vi "ReadSpetroFile.vi"(1 "本次文件名":string) -> ()   [LabVIEW 2018]
uses:
  Init/AllPath.vi
  <vilib>/Utility/file.llb/Read Delimited Spreadsheet (string).vi
  HistoryFile.vi
panel:
  out "波形":cluster{"数组":dbl[], "数组":dbl[]}
  out "脉宽":string
  out "中心波长":string
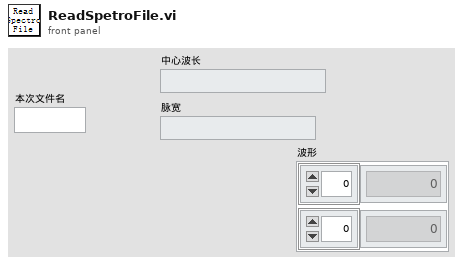
[diagram p1: front panel]
types:
  T1 = cluster{"能量/功率":path, " 示波器":path, " 光谱仪":path, "偏振":path, "近远场":cluster{" 近场图片":path, " 远场图片":path, "发散角数据":path}, "参数":path, " 基路径":path, "文件名信息":path, "输出模板路径":path, "输出报告路径":path, "位置信息路径":path}
  T2 = cluster{"中心波长":string, " 谱宽":string, " 中心波长Uint":string, " 谱宽 Uint":string, "波形":cluster{"数组":dbl[], "数组":dbl[]}}
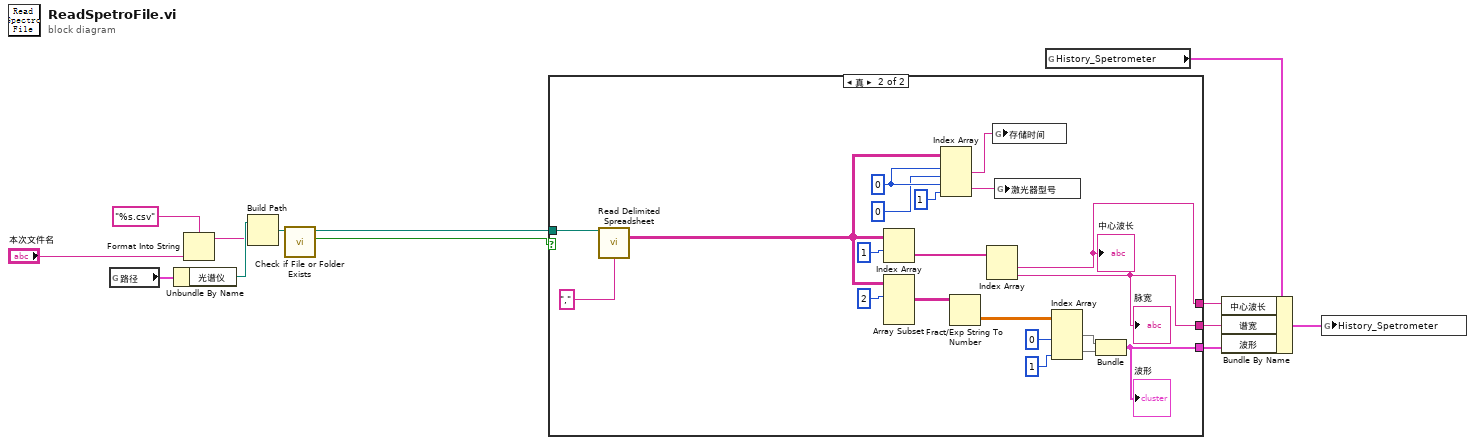
[diagram p0: block diagram]
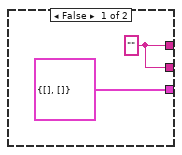
[diagram p2: hidden frame]
diagram:
  n1 = global read "AllPath.vi" "路径"() -> (w13:T1)
  n2 = Unbundle By Name(w13) -> ("光谱仪"=w12:path)
  n3 = Format Into String(format string="%s.csv" ("格式字符串"), "本次文件名") -> (resulting string=w9:string)  [unwired: 2 in, 1 out]
  n4 = Build Path(base path=w12, name or relative path=w9) -> (appended path=w3:path)
  n5 = call <vilib>:"Check if File or Folder Exists.vi"("path"=w3) -> ("file or folder exists?"=w1:bool, "dup path"=w2:path)  [unwired: 8 in, 1 out]
  n6 = case shown="真" w1 {
    tunnel: w2 -> [_ w35]
    tunnel: [w15 w24] -> w7
    tunnel: [w15 w23] -> w6
    tunnel: [cluster{dbl[], dbl[]} {[], []} w22] -> w5
    frame False {
      w15 = ""
    }
    frame True {
      w20 = 0 ("索引 (行)")
      n7 = call-poly <vilib>:"Read Delimited Spreadsheet.vi"("file path (dialog if empty)"=w35, "delimiter (\\t)"="," ("delimiter (\\t)")) -> ("all rows"=w21:string[][])  [unwired: 8 in, 5 out]
      n8 = Index Array(array=w21, index (row)=1 ("索引 (行)")) -> (element=w32:string[])  [unwired: 1 in]
      n9 = Array Subset(array=w21, index (row)=2 ("索引")) -> (w30:string[][])  [unwired: 3 in]
      n10 = Index Array(array=w21, index (row) #1=w20, index (col) #1=0 ("禁用的索引 (列)"), index (row) #2=w20, index (col) #2=1 ("禁用的索引 (列)")) -> (element #1=w17:string, element #2=w16:string)
      n11 = Fract/Exp String To Number(string=w30) -> (number=w29:dbl[][])  [unwired: 3 in, 1 out]
      n12 = Index Array(array=w32) -> (element #1=w24:string, element #2=w23:string)  [unwired: 2 in]
      "中心波长" <- w24
      "脉宽" <- w23
      n13 = global write "HistoryFile.vi" "存储时间"(w17) -> ()
      n14 = global write "HistoryFile.vi" "激光器型号"(w16) -> ()
      n15 = Index Array(array=w29, index (col) #1=0 ("禁用的索引 (列)"), index (col) #2=1 ("索引 (列)")) -> (element #1=w26:dbl[], element #2=w25:dbl[])  [unwired: 2 in]
      n16 = Bundle(w26, w25) -> (w22:cluster{dbl[], dbl[]})  [unwired: 1 in]
      "波形" <- w22
    }
  }
  n17 = global read "HistoryFile.vi" "History_Spetrometer"() -> (w8:T2)
  n18 = Bundle By Name(cluster=w8, "中心波长"=w7, "谱宽"=w6, "波形"=w5) -> (w4:T2)
  n19 = global write "HistoryFile.vi" "History_Spetrometer"(w4) -> ()
